vi "Controller Deadband Increaced Limit for Demos.vi"(7 "Input":dbl) -> (6 "Output":dbl)   [LabVIEW 2017]
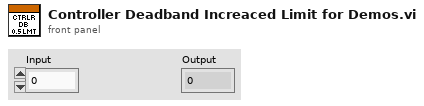
[diagram p1: front panel]
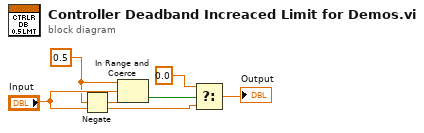
[diagram p0: block diagram]
diagram:
  w1 = 0.5 ("upper limit")
  n1 = Negate(x=w1) -> (-x=w2:dbl)
  n2 = In Range and Coerce(upper limit=w1, x="Input", lower limit=w2) -> (In Range?=w3:bool)  [unwired: 1 out]
  n3 = Select(t=0.0, s=w3, f="Input") -> (s? t:f=→"Output":dbl)
